vi "-Send_And_Receive_Message.vi"(8 "error in (no error)":errorcluster, 10 "Message To Send":string, 11 "Postgres Connector In":refnum<class "Postgres Connector.lvclass">) -> (0 "error out":errorcluster, 3 "Postgres Connector Out":refnum<class "Postgres Connector.lvclass">)   [LabVIEW 2020, in "Postgres Connector.lvclass"]
doc: "This send the message of the client to the Postgres database using TCP, then read the answer from the database."
uses:
  Postgres Connector.lvclass
  Postgres Connector.lvclass/Postgres Connector.ctl
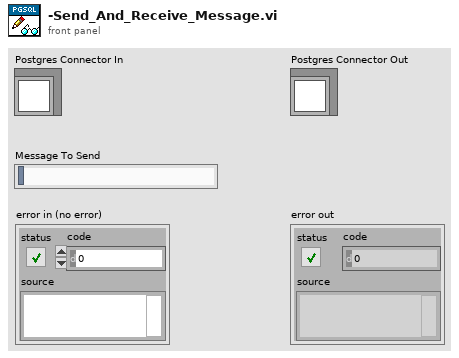
[diagram p1: front panel]
types:
  T1 = enum16{"Standard", "Buffered", "CRLF", "Immediate"}
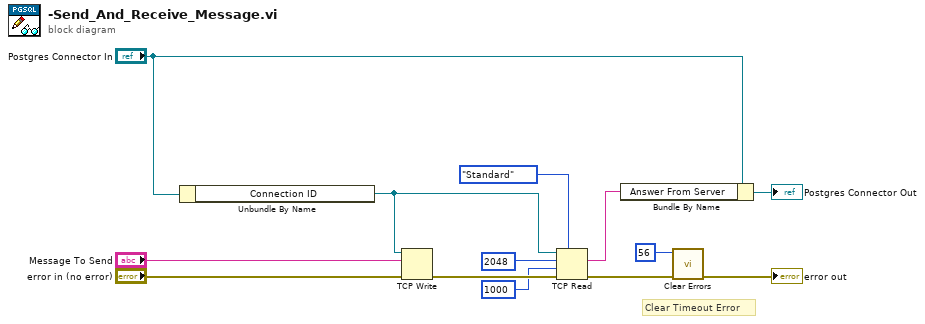
[diagram p0: block diagram]
diagram:
  # "Clear Timeout Error"
  n1 = Unbundle By Name("Postgres Connector In") -> ("Connection ID"=w1:refnum<k5>)
  n2 = TCP Write(connection ID=w1, data in="Message To Send", error in (no error)="error in (no error)") -> (error out=w7:errorcluster)  [unwired: 1 in, 2 out]
  n3 = TCP Read(connection ID=w1, bytes to read=2048, error in (no error)=w7, 7:T1."Standard" ("mode (standard)"), 9:1000 ("timeout ms (25000)")) -> (data out=w8:string, error out=w6:errorcluster)  [unwired: 1 out]
  n4 = Bundle By Name(cluster="Postgres Connector In", "Answer From Server"=w8) -> (→"Postgres Connector Out":refnum<class "Postgres Connector.lvclass">)
  n5 = call <vilib>:"Clear Errors.vi"("error in (no error)"=w6, "specific error code to clear (0: all)"=56) -> ("error out"=→"error out":errorcluster)  [unwired: 4 in, 1 out]
